vi "Log shot data.vi"(8 "error in (no error)":errorcluster, 9 "Spreadsheet header string":string, 10 "Spreadsheet shot string":string, 11 "Log file folder":path=path "C:/Data/Shot Log.txt") -> (0 "error out":errorcluster, 3 "path":path)   [LabVIEW 2015]
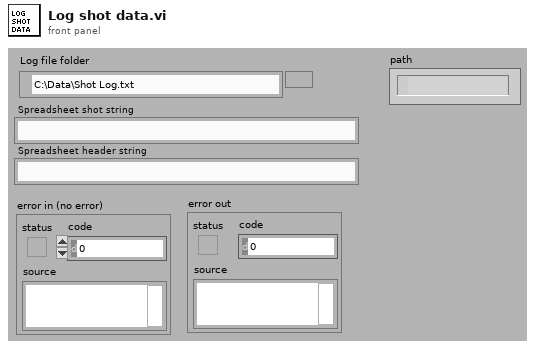
[diagram p1: front panel]
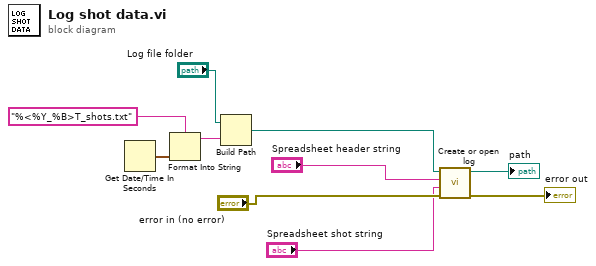
[diagram p0: block diagram]
diagram:
  n1 = Get Date/Time In Seconds() -> (seconds since 1Jan1904=w10:timestamp)
  n2 = Format Into String(format string="%<%Y_%B>T_shots.txt", w10) -> (resulting string=w8:string)  [unwired: 2 in, 1 out]
  n3 = Build Path(base path="Log file folder", name or relative path=w8) -> (appended path=w6:path)
  n4 = call "Create or open log.vi"("error in (no error)"="error in (no error)", "Log string"="Spreadsheet shot string", "Spreadsheet header string"="Spreadsheet header string", "appended path"=w6) -> ("error out"=→"error out":errorcluster, "path"=→"path":path)  [unwired: 6 in]
